vi "Cable Parameter KaaKbbKd.vi"(0 "VISA resource name":refnum<visa-resource-name>, 1 "Cable Length (0:0)":enum16{"0m", "1m", "2m", "4m"}(ring), 2 "Frequency (20)":dbl=20.0 min=20.0 max=1000000.0 format="%.2f", 5 "Voltage Level (1.0)":dbl=1.0 min=0.005 max=20.0 format="%.3f", 7 "Impedance Z (10m)":dbl=0.01 min=0.01 max=100000000.0 format="%^.2e", 9 "Ka":dbl format="%.3f", 11 "error in (no error)":errorcluster) -> (4 "VISA resource name out":refnum<visa-resource-name>, 6 "Kaa":dbl format="%.3f", 8 "Kd":dbl format="%.3f", 10 "Kbb":dbl format="%.3f", 15 "error out":errorcluster)   [LabVIEW 2015, in "Agilent 428X Series.lvlib"]
doc: "This Vi calculate the cable parameters : Kaa, Kbb, and Kd. These three parameters will be used for calculating the relative accuracy Ae.\nKaa:\n Cable Length\n 0m 1m 2m \n<=2 Vrms 0 0 Ka/2 \n>2 Vrms 0 (2*10E-3 * f^2)/Z (1+5*f^2)*10E-3/Z \n 4m\n<=2Vrms Ka\n>2Vrms (2+10*f^2)*10E-3/Z \n\nKbb: \n Cable Length\n 0m 1m 2m 4m \nf<=100 1 1+5*f 1+10*f 1+20*f\n100k<f<300K 1 1+2*f 1+4*f 1+8*f\n300K<f<1M 1 1+0.5f 1+1*f 1+2*f\n\nKd:\n Cable Length \n 1m 2m 3m\n<=2Vrms 2.5*10E-4*a 5*10E-4*a 1*10E-3*a\n>2Vrms 2.5*10E-3*b 5*10E-3*b 1*10E-2*b\n\na=1+50*f\nb=1+16*f\n\nDisclaimer: All accuracy calculation VI's are not part of the original \n driver. They are provided for supplementry purpose only.\n If user desires very high accuracy data, please do or \n check the calculation seperately."
uses:
  <instrlib>/Agilent 428X Series/Agilent 428X Series.lvlib
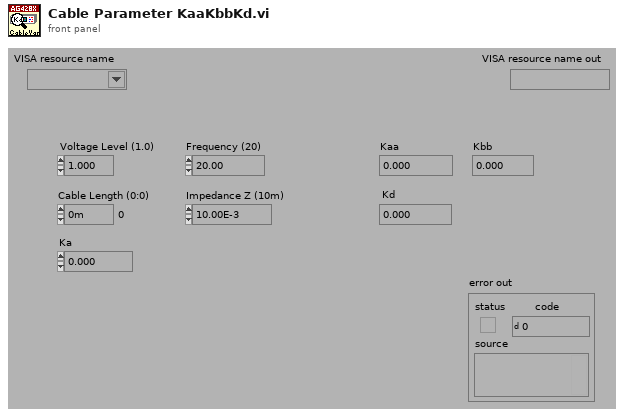
[diagram p1: front panel]
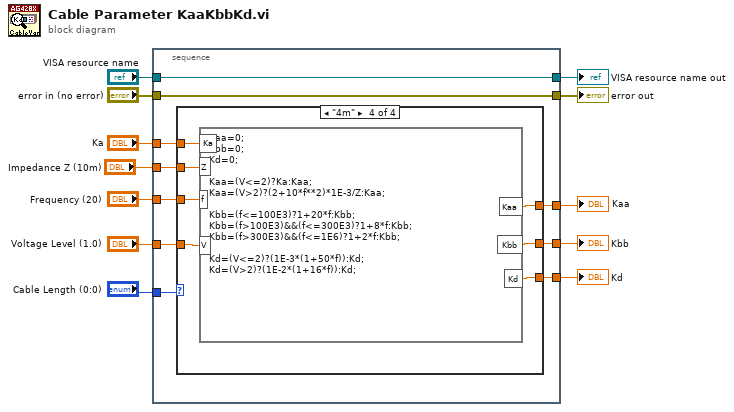
[diagram p0: block diagram]
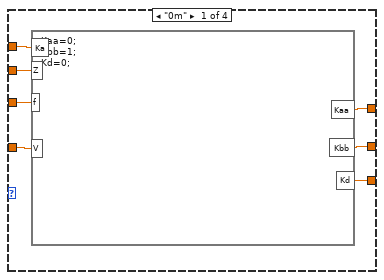
[diagram p2: hidden frame]
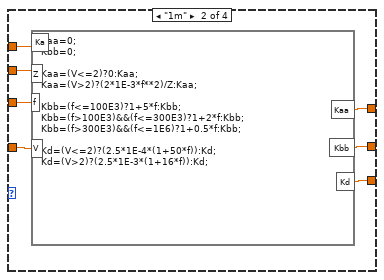
[diagram p3: hidden frame]
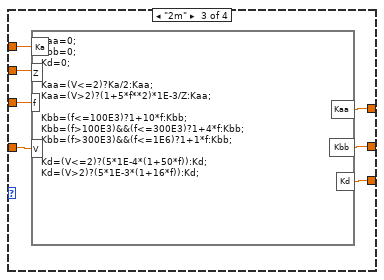
[diagram p4: hidden frame]
diagram:
  n1 = stacked-sequence {
    tunnel: "VISA resource name" -> [w22]
    tunnel: [w22] -> w11
    tunnel: [w21] -> w10
    tunnel: "error in (no error)" -> [w21]
    tunnel: "Cable Length (0:0)" -> [w20]
    tunnel: "Voltage Level (1.0)" -> [w19]
    tunnel: "Frequency (20)" -> [w18]
    tunnel: [w17] -> w5
    tunnel: [w16] -> w4
    tunnel: [w15] -> w3
    tunnel: "Ka" -> [w14]
    tunnel: "Impedance Z (10m)" -> [w13]
    frame #0 {
      n2 = case shown="\"4m\"" w20 {
        tunnel: w19 -> [w29 w36 w43 w50]
        tunnel: w18 -> [w28 w35 w42 w49]
        tunnel: [w27 w34 w41 w48] -> w17
        tunnel: [w26 w33 w40 w47] -> w16
        tunnel: [w25 w32 w39 w46] -> w15
        tunnel: w14 -> [w24 w31 w38 w45]
        tunnel: w13 -> [w23 w30 w37 w44]
        frame "0m" {
          n3 = formula code="Kaa=0;\nKbb=1;\nKd=0;"("V"=w29, "f"=w28, "Ka"=w24, "Z"=w23) -> ("Kaa"=w27:dbl, "Kbb"=w26:dbl, "Kd"=w25:dbl)
        }
        frame "1m" {
          n4 = formula code="Kaa=0;\nKbb=0;\n\nKaa=(V<=2)?0:Kaa;\nKaa=(V>2)?(2*1E-3*f**2)/Z:Kaa;\n\nKbb=(f<=100E3)?1+5*f:Kbb;\nKbb=(f>100E3)&&(f<=300E3)?1+2*f:Kbb;\nKbb=(f>300E3)&&(f<=1E6)?1+0.5*f:Kbb;\n\nKd=(V<=2)?(2.5*1E-4*(1+50*f)):Kd;\nKd=(V>2)?(2.5*1E-3*(1+16*f)):Kd;"("V"=w36, "f"=w35, "Ka"=w31, "Z"=w30) -> ("Kaa"=w34:dbl, "Kbb"=w33:dbl, "Kd"=w32:dbl)
        }
        frame "2m" {
          n5 = formula code="Kaa=0;\nKbb=0;\nKd=0;\n\nKaa=(V<=2)?Ka/2:Kaa;\nKaa=(V>2)?(1+5*f**2)*1E-3/Z:Kaa;\n\nKbb=(f<=100E3)?1+10*f:Kbb;\nKbb=(f>100E3)&&(f<=300E3)?1+4*f:Kbb;\nKbb=(f>300E3)&&(f<=1E6)?1+1*f:Kbb;\n\nKd=(V<=2)?(5*1E-4*(1+50*f)):Kd;\nKd=(V>2)?(5*1E-3*(1+16*f)):Kd;"("V"=w43, "f"=w42, "Ka"=w38, "Z"=w37) -> ("Kaa"=w41:dbl, "Kbb"=w40:dbl, "Kd"=w39:dbl)
        }
        frame "4m" {
          n6 = formula code="Kaa=0;\nKbb=0;\nKd=0;\n\nKaa=(V<=2)?Ka:Kaa;\nKaa=(V>2)?(2+10*f**2)*1E-3/Z:Kaa;\n\nKbb=(f<=100E3)?1+20*f:Kbb;\nKbb=(f>100E3)&&(f<=300E3)?1+8*f:Kbb;\nKbb=(f>300E3)&&(f<=1E6)?1+2*f:Kbb;\n\nKd=(V<=2)?(1E-3*(1+50*f)):Kd;\nKd=(V>2)?(1E-2*(1+16*f)):Kd;"("V"=w50, "f"=w49, "Ka"=w45, "Z"=w44) -> ("Kaa"=w48:dbl, "Kbb"=w47:dbl, "Kd"=w46:dbl)
        }
      }
    }
  }
  "VISA resource name out" <- w11
  "error out" <- w10
  "Kaa" <- w5
  "Kbb" <- w4
  "Kd" <- w3
